vi "Verify Class Roster as JSON.vi"(8 "error in":errorcluster) -> (0 "error out":errorcluster)   [LabVIEW 2020, in "Caraya Extension Tests.lvclass"]
uses:
  Caraya Extension Tests.lvclass
  <vilib>/addons/_JKI Toolkits/Caraya/classes/Test/Test.lvclass
  Source/Extensions/Caraya.Extension/Caraya.Extension.lvlib
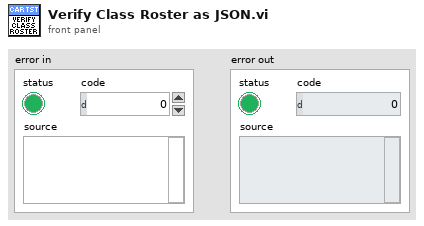
[diagram p1: front panel]
types:
  T1 = cluster{"Subject":string, "Teacher":cluster{"First Name":string, "Last Name":string}, "Assignments":cluster{"Description":string, "Grades":map{cluster{"First Name":string, "Last Name":string}, i32}}[], "Roster":cluster{"First Name":string, "Last Name":string}[]}
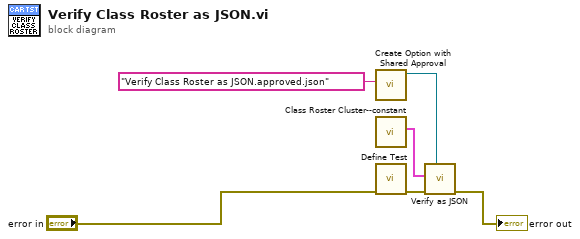
[diagram p0: block diagram]
diagram:
  n1 = call "Create Option with Shared Approval.vi"("Filename"="Verify Class Roster as JSON.approved.json") -> ("Options outs"=w1:refnum<class "Options.lvclass">)  [unwired: 10 in]
  n2 = call "Class Roster Cluster--constant.vi"() -> ("Class Roster"=w3:T1)  [unwired: 11 in]
  n3 = call <vilib>:"Define Test.vi"("error in (no error)"="error in") -> ("error out"=w6:errorcluster)  [unwired: 9 in, 1 out]
  n4 = call "Verify as JSON.vi"("Options"=w1, "error in"=w6, "Anything"=w3) -> ("error out"=→"error out":errorcluster)  [unwired: 7 in, 1 out]
